vi "User Info.vi"(11 "User Entrence":string) -> ()   [LabVIEW 2020]
uses:
  <vilib>/addons/database/Connection.llb/Conn ObjectReference.ctl
  <vilib>/Utility/error.llb/whitespace.ctl
  <vilib>/addons/database/Connection.llb/DB Tools Open Connec (String).vi
  <vilib>/addons/database/Connection.llb/Conn Execute.vi
  <vilib>/addons/database/Recordset.llb/Rec Fetch Recordset Data (R).vi
  <vilib>/addons/database/Recordset.llb/Rec Destroy - Connection.vi
  <vilib>/addons/database/_DB Variant To Data/Database Variant To Data.xnode
  <vilib>/addons/database/NI_Database_API.lvlib
panel:
  in  "Back":bool
  in  "Tab Control":T1(tab)
  in  "User_Name 7":string caption="用户名"
  in  "User_Password 2":string caption="密    码"
  in  "Login":bool
  in  "Remember Passwrod":bool caption="记住密码"
  in  "Remember User Name":bool caption="记住用户名"
  in  "User Regist":bool
  in  "User Change":bool caption="切换用户"
  in  "User Manage":bool
  in  "Change Password":bool
  in  "User_Right 2":u16(ring) caption="权    限" items=["Manufacturer", "Foreman", "Professional", "Operator"]
  in  "User_Name 4":string caption="用户名"
  in  "Confirm Password 2":string caption="确认密码"
  in  "New Password 2":string caption="新  密  码"
  in  "Last Password":string caption="旧  密  码"
  in  "User Change Btn":bool
  in  "User_Name 3":string caption="用  户  名"
  in  "User_Password":string caption="密        码"
  in  "User_Name":string caption="用  户  名"
  in  "Ok":bool
  in  "User List":i32(listbox)
  in  "User_Right":u16(ring) caption="权        限" items=["Manufacturer", "Foreman", "Professional", "Operator"]
  in  "Confirm Password":string caption="确认密码"
  in  "New Password":string caption="密        码"
  in  "Ok 2":bool
  in  "User_Name 2":string caption="用  户  名"
  in  "User_Right 3":u16(ring) caption="权        限" items=["Manufacturer", "Foreman", "Professional", "Operator"]
  in  "Confirm Password 3":string caption="确认密码"
  in  "New Password 3":string caption="新  密  码"
  in  "Ok 4":bool
  in  "User_Name 5":string caption="用  户  名"
  in  "Confirm Password 4":string caption="确认密码"
  in  "New Password 4":string caption="密        码"
  in  "Regist":bool
  in  "User_Name 6":string caption="用  户  名"
  out "Title":string
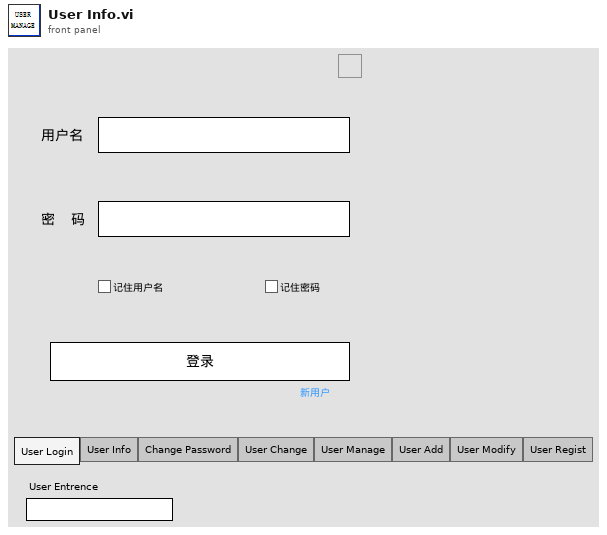
[diagram p1: front panel]
types:
  T1 = enum32{"User Login", "User Info", "Change Password", "User Change", "User Manage", "User Add", "User Modify", "User Regist"}
  T2 = typedef "NI_Database_API.lvlib/Conn ObjectReference.ctl" = refnum<k1>
  T3 = cluster{"DB Ref In":T2, "User Name":string, "User Password":string, "User Right":i32, "Language":string, "Current Page":string, "Tab Control":refnum<vi>, "Remember Name":bool, "Remember PW":bool}
  T4 = enum32{"Invalid", "Standard", "Closed", "Hidden", "Minimized", "Maximized"}
  T5 = cluster{"User Name":string, "User Right":i32, "User Password":string, string, string, "seconds since 1Jan1904":timestamp}
  T6 = typedef "whitespace.ctl" = u16
  T7 = typedef "NI_Database_API.lvlib/Rec ObjectReference.ctl" = refnum<k1>
  T8 = typedef "LVPoint32TypeDef.ctl" = cluster{"Horizontal":i32, "Vertical":i32}
  T9 = typedef "LVRowAndColumnTypeDef.ctl" = cluster{"Row":i32, "Column":i32}
  T10 = enum32{"invalid app kind", "Development System", "Run Time System", "Student Edition", "Embedded LabVIEW", "Evaluation", "Custom"}
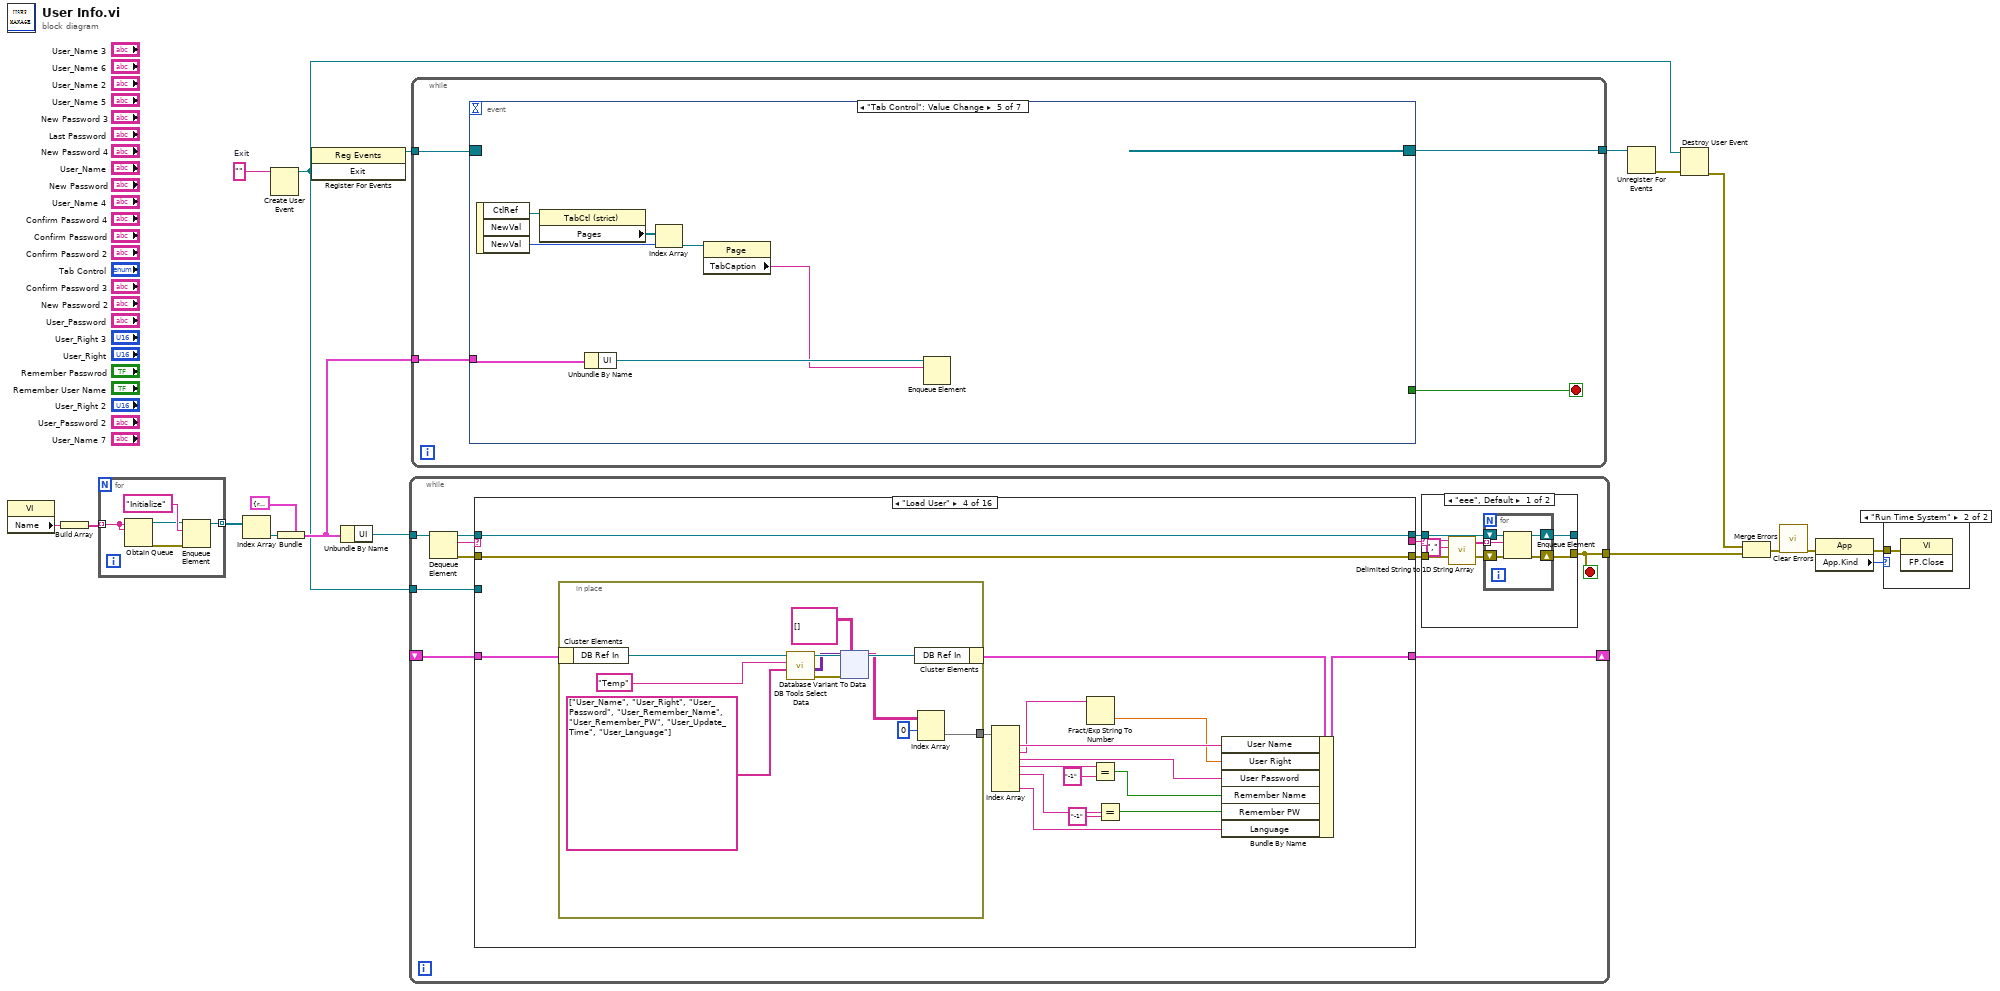
[diagram p0: block diagram]
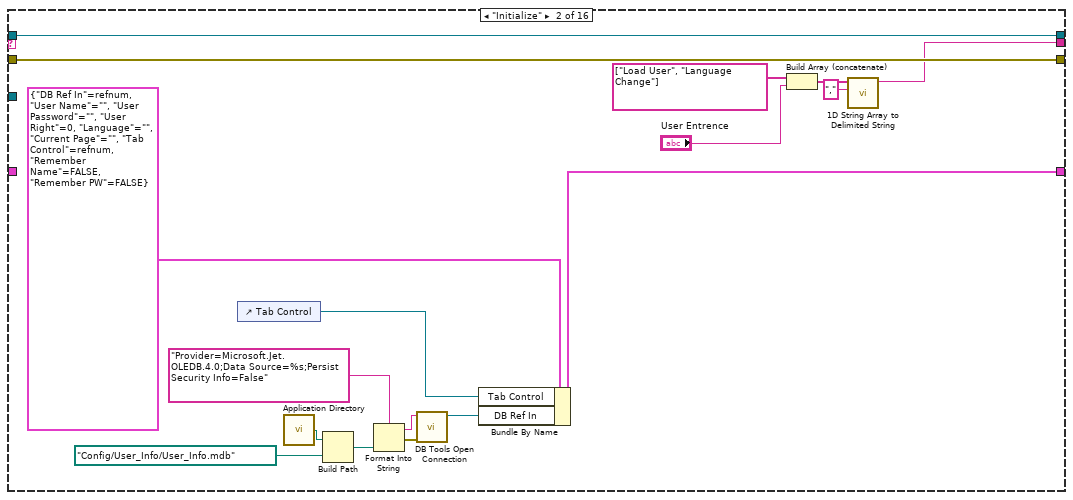
[diagram p5: hidden frame]
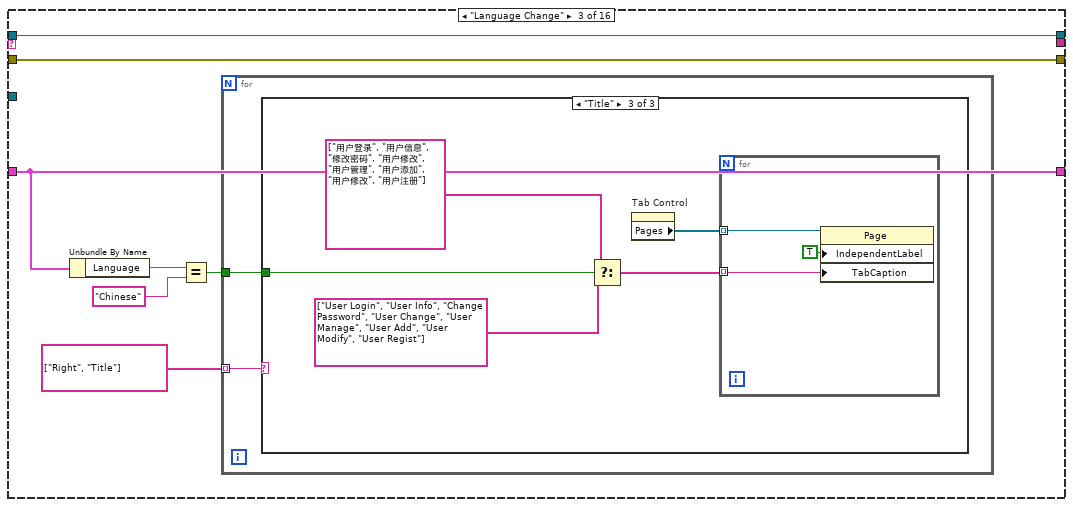
[diagram p6: hidden frame]
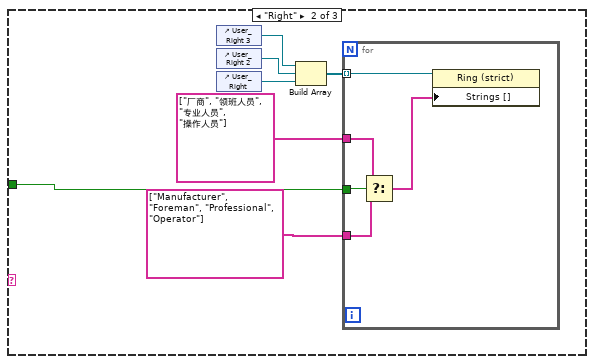
[diagram p8: hidden frame]
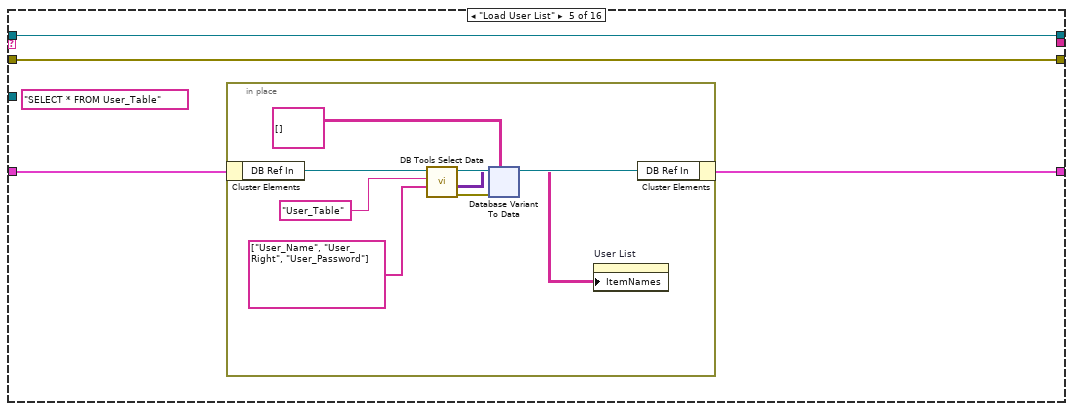
[diagram p9: hidden frame]
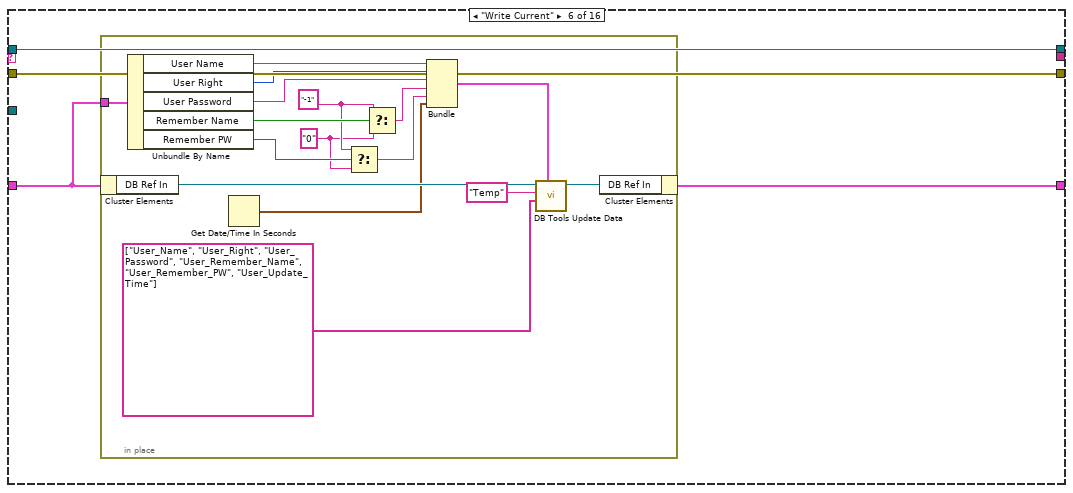
[diagram p10: hidden frame]
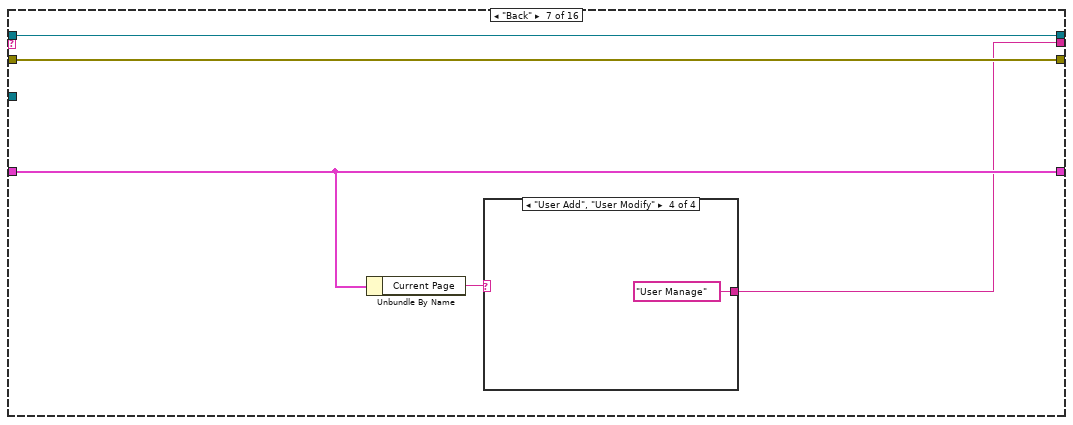
[diagram p11: hidden frame]
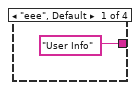
[diagram p12: hidden frame]
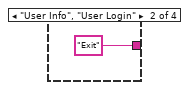
[diagram p13: hidden frame]
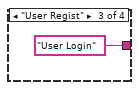
[diagram p14: hidden frame]
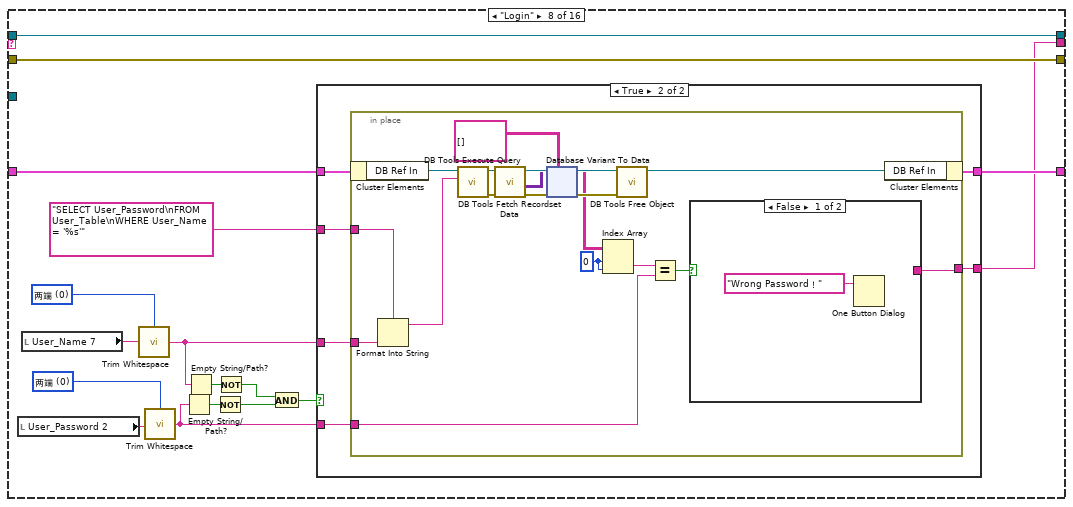
[diagram p15: hidden frame]
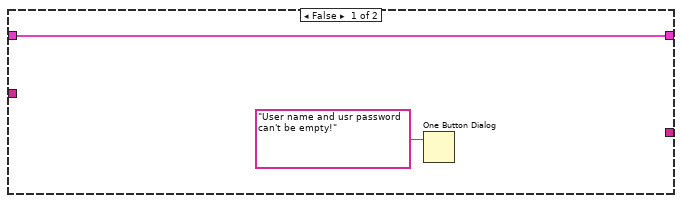
[diagram p16: hidden frame]
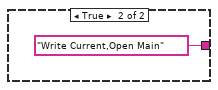
[diagram p17: hidden frame]
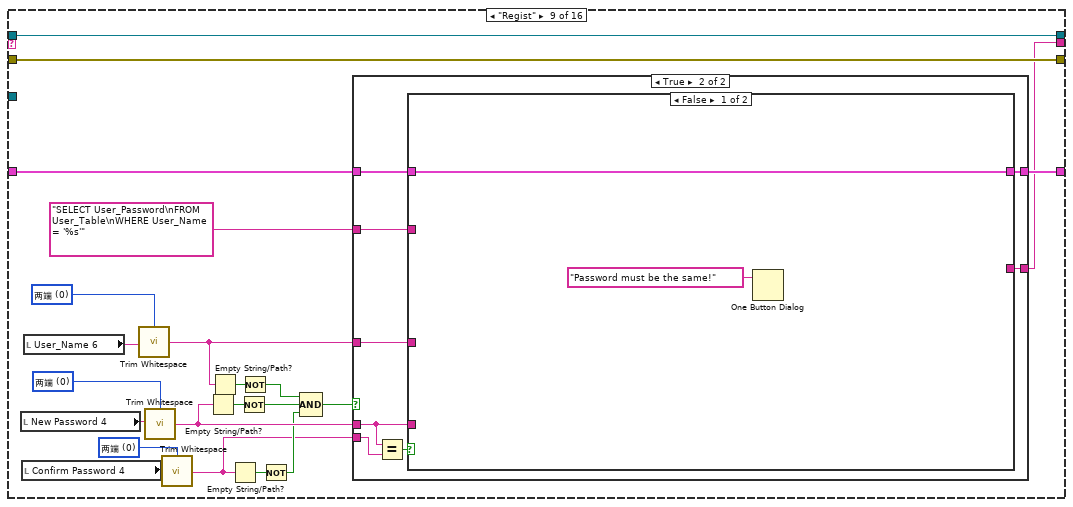
[diagram p18: hidden frame]
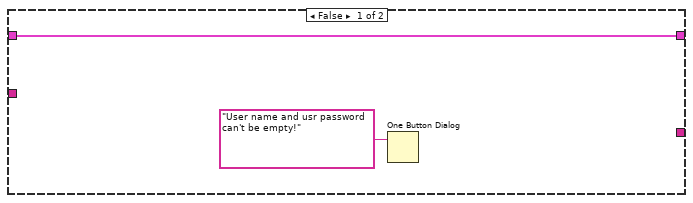
[diagram p19: hidden frame]
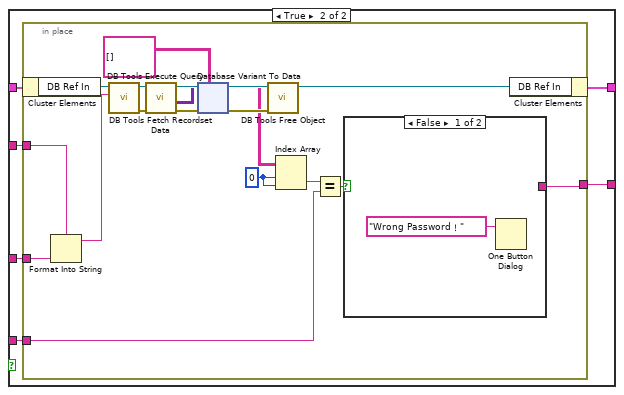
[diagram p20: hidden frame]
diagram:
  w3 = ""  # Exit
  n1 = property class="VI"() -> ("Name"=w13:string)  [unwired: 2 in, 2 out]
  n2 = Build Array(w13) -> (w14:string[])
  n3 = for {
    tunnel: w14 -> [w19] mode=indexing
    tunnel: [w20] -> w8 mode=indexing
    n4 = Obtain Queue(name (unnamed)=w19, element data type=w19) -> (queue out=w22:refnum<queue>, error out=w21:errorcluster)  [unwired: 3 in, 1 out]
    n5 = Enqueue Element(queue=w22, element="Initialize" ("元素"), error in (no error)=w21) -> (queue out=w20:refnum<queue>)  [unwired: 1 in, 2 out]
  }
  n6 = Index Array(array=w8) -> (element=w11:refnum<queue>)  [unwired: 1 in]
  n7 = Create User Event(user event datatype=w3) -> (user event=w7:refnum<user-event>)  [unwired: 1 in, 1 out]
  n8 = Bundle(cluster=cluster{"UI":refnum<queue>} {"UI"=refnum}, "UI"=w11) -> (w12:cluster{"UI":refnum<queue>})
  n9 = register-events(w7) -> (reference out=w4:refnum<event-registration>)  [unwired: 2 in, 1 out]
  n10 = Unbundle By Name(w12) -> ("UI"=w9:refnum<queue>)
  n11 = while {
    tunnel: w9 -> [w34]
    tunnel: [w24] -> w16
    shift-right: [w28] -> _
    shift-left: _ -> [w27]
    tunnel: w7 -> [w26]
    stop <- w24 stop-if-true
    n12 = Dequeue Element(queue=w34) -> (queue out=w33:refnum<queue>, element=w25:string, error out=w30:errorcluster)  [unwired: 2 in, 1 out]
    n13 = case shown="\"Load User\"" w25 {
      selector: w25 -> [_ _ _ _ _ _ _ _ _ _ _ _ _ w469 w524 _]
      tunnel: w33 -> [w51 w59 w75 w114 w172 w228 w249 w270 w364 w456 w459 w462 w465 w474 w529 w535]
      tunnel: [w51 w59 w75 w114 w172 w228 w249 w270 w364 w456 w459 w462 w465 w474 w528 w535] -> w32
      tunnel: [w50 w58 w74 w113 w171 w227 w248 w269 w363 w455 w458 w461 w464 w473 w527 w532] -> w31
      tunnel: w30 -> [w50 w58 w74 w113 w171 w227 w248 w269 w363 w455 w458 w461 w464 w473 w526 w534]
      tunnel: [_ w52 _ _ _ _ w245 w257 w352 "Exit" ("Message") _ _ _ w467 "Quit" ("Message") _] -> w29
      tunnel: [w49 w61 w73 w111 w169 w226 w247 w260 w354 w454 w457 w460 w463 w468 w531 w533] -> w28
      tunnel: w27 -> [w49 _ w73 w112 w170 w225 w247 w261 w355 w454 w457 w460 w463 w472 w531 w533]
      tunnel: w26 -> [_ _ _ _ _ _ _ _ _ _ _ _ _ _ w525 _]
      frame "eee", Default {
      }
      frame "Initialize" {
        n14 = control-ref of="Tab Control"() -> (w55:refnum<vi>)
        n15 = call <vilib>:"Application Directory.vi"() -> ("Application Directory"=w64:path)
        n16 = Build Path(base path=w64, name or relative path=path "Config/User_Info/User_Info.mdb" ("名称或相对路径")) -> (appended path=w62:path)
        n17 = Format Into String(format string="Provider=Microsoft.Jet.OLEDB.4.0;Data Source=%s;Persist Security Info=False", w62) -> (resulting string=w66:string, error out=w65:errorcluster)  [unwired: 2 in]
        n18 = call-poly <vilib>:"DB Tools Open Connection.vi"("error in (no error)"=w65, "connection information"=w66) -> ("connection reference"=w60:T2)  [unwired: 6 in, 1 out]
        n19 = Bundle By Name(cluster=T3 {"DB Ref In"=refnum, "User Name"="", "User Password"="", "User Right"=0, "Language"="", "Current Page"="", "Tab Control"=refnum, "Remember Name"=FALSE, "Remember PW"=FALSE} ("Data"), "Tab Control"=w55, "DB Ref In"=w60) -> (w61:T3)
        n20 = Build Array (concatenate)(string[] ["Load User", "Language Change"], "User Entrence") -> (w54:string[])
        n21 = call <vilib>:"1D String Array to Delimited String.vi"("delimiter"=",", "string array"=w54) -> ("delimited string"=w52:string)  [unwired: 9 in]
      }
      frame "Language Change" {
        n22 = Unbundle By Name(w73) -> ("Language"=w72:string)
        n23 = Equal?(x=w72, y="Chinese") -> (x = y?=w69:bool)
        n24 = for {
          tunnel: string[] ["Right", "Title"] -> [w77] mode=indexing
          tunnel: w69 -> [w76]
          n25 = case shown="\"Title\"" w77 {
            tunnel: w76 -> [_ w78 w94]
            frame "eee", Default {
            }
            frame "Right" {
              n26 = control-ref of="User_Right 3"() -> (w81:refnum<vi>)
              n27 = control-ref of="User_Right 2"() -> (w82:refnum<vi>)
              n28 = control-ref of="User_Right"() -> (w83:refnum<vi>)
              n29 = Build Array(w81, w82, w83) -> (w84:refnum<vi>[])
              n30 = for {
                tunnel: w84 -> [w89] mode=indexing
                tunnel: string[] ["厂商", "领班人员", "专业人员", "操作人员"] -> [w88]
                tunnel: string[] ["Manufacturer", "Foreman", "Professional", "Operator"] -> [w87]
                tunnel: w78 -> [w85]
                n31 = Select(t=w88, s=w85, f=w87) -> (s? t:f=w86:string[])
                n32 = property class="Ring (strict)"(reference=w89, "Strings []"=w86) -> ()  [unwired: 1 in, 2 out]
              }
            }
            frame "Title" {
              n33 = Select(t=string[] ["用户登录", "用户信息", "修改密码", "用户修改", "用户管理", "用户添加", "用户修改", "用户注册"], s=w94, f=string[] ["User Login", "User Info", "Change Password", "User Change", "User Manage", "User Add", "User Modify", "User Regist"]) -> (s? t:f=w90:string[])
              n34 = property on="Tab Control" class="TabCtl (strict)"() -> ("Pages"=w91:refnum<vi>[])  [unwired: 2 in, 2 out]
              n35 = for {
                tunnel: w91 -> [w97] mode=indexing
                tunnel: w90 -> [w96] mode=indexing
                n36 = property class="Page"(reference=w97, "IndependentLabel"=TRUE ("独立标签"), "TabCaption"=w96) -> ()  [unwired: 1 in, 2 out]
              }
            }
          }
        }
      }
      frame "Load User" {
        n37 = in-place {
          in-place-border: [w115] -> w109
          n38 = in-place-cluster #1(w112) -> ("DB Ref In"=w124:T2)
          n39 = call <vilib>:"DB Tools Select Data.vi"("columns"=string[] ["User_Name", "User_Right", "User_Password", "User_Remember_Name", "User_Remember_PW", "User_Update_Time", "User_Language"], "table"="Temp", "connection reference"=w124) -> ("error out"=w118:errorcluster, "data"=w120:variant[][], "connection reference out"=w123:T2)  [unwired: 3 in]
          n40 = xnode "Database Variant To Data"("database variant"=w120, "error in (no error)"=w118, "type"=string[][] []) -> ("data"=w117:string[][])  [unwired: 1 out]
          n41 = in-place-cluster #1("DB Ref In"=w123) -> (w110:T3)
          n42 = Index Array(array=w117, index (row)=0 ("索引 (行)")) -> (element=w115:string[])  [unwired: 1 in]
        }
        n43 = Index Array(array=w109) -> (element #1=w108:string, element #2=w99:string, element #3=w107:string, element #4=w106:string, element #5=w102:string, element #7=w100:string)  [unwired: 7 in, 1 out]
        n44 = Fract/Exp String To Number(string=w99) -> (number=w98:dbl)  [unwired: 3 in, 1 out]
        n45 = Equal?(x=w106, y="-1") -> (x = y?=w104:bool)
        n46 = Equal?(x=w102, y="-1") -> (x = y?=w101:bool)
        n47 = Bundle By Name(cluster=w110, "User Name"=w108, "User Right"=w98, "User Password"=w107, "Remember Name"=w104, "Remember PW"=w101, "Language"=w100) -> (w111:T3)
      }
      frame "Load User List" {
        (unwired) "SELECT * FROM User_Table" ("SQL query")
        n48 = in-place {
          n49 = in-place-cluster #2(w170) -> ("DB Ref In"=w180:T2)
          n50 = call <vilib>:"DB Tools Select Data.vi"("columns"=string[] ["User_Name", "User_Right", "User_Password"] ("table"), "table"="User_Table", "connection reference"=w180) -> ("error out"=w176:errorcluster, "data"=w175:variant[][], "connection reference out"=w179:T2)  [unwired: 3 in]
          n51 = xnode "Database Variant To Data"("database variant"=w175, "error in (no error)"=w176, "type"=string[][] []) -> ("data"=w173:string[][])  [unwired: 1 out]
          n52 = property on="User List" class="MCListbox (strict)"("ItemNames"=w173) -> ()  [unwired: 2 in, 2 out]
          n53 = in-place-cluster #2("DB Ref In"=w179) -> (w169:T3)
        }
      }
      frame "Write Current" {
        n54 = in-place {
          in-place-border: w225 -> [w241]
          w230 = "0"
          w231 = "-1"
          n55 = in-place-cluster #3(w225) -> ("DB Ref In"=w244:T2)
          n56 = Unbundle By Name(w241) -> ("User Name"=w240:string, "User Right"=w239:i32, "User Password"=w238:string, "Remember Name"=w235:bool, "Remember PW"=w233:bool)
          n57 = Get Date/Time In Seconds() -> (seconds since 1Jan1904=w229:timestamp)
          n58 = Select(t=w231, s=w233, f=w230) -> (s? t:f=w232:string)
          n59 = Select(t=w231, s=w235, f=w230) -> (s? t:f=w234:string)
          n60 = Bundle("User Name"=w240, "User Right"=w239, "User Password"=w238, w234, w232, "seconds since 1Jan1904"=w229) -> (w237:T5)  [unwired: 1 in]
          n61 = call <vilib>:"DB Tools Update Data.vi"("data"=w237, "columns"=string[] ["User_Name", "User_Right", "User_Password", "User_Remember_Name", "User_Remember_PW", "User_Update_Time"], "table"="Temp", "connection reference"=w244) -> ("connection reference out"=w243:T2)  [unwired: 6 in, 1 out]
          n62 = in-place-cluster #3("DB Ref In"=w243) -> (w226:T3)
        }
      }
      frame "Back" {
        n63 = Unbundle By Name(w247) -> ("Current Page"=w246:string)
        n64 = case shown="\"User Add\", \"User Modify\"" w246 {
          tunnel: ["User Info" "Exit" "User Login" "User Manage"] -> w245
          frame "eee", Default {
          }
          frame "User Info", "User Login" {
          }
          frame "User Regist" {
          }
          frame "User Add", "User Modify" {
          }
        }
      }
      frame "Login" {
        w267 = T6 0 items=["两端", "字符串首端", "字符串末端"] ("location (both)")
        w268 = T6 0 items=["两端", "字符串首端", "字符串末端"] ("location (both)")
        n65 = local read "User_Password 2"() -> (w254:string)
        n66 = local read "User_Name 7"() -> (w255:string)
        n67 = call <vilib>:"Trim Whitespace.vi"("string"=w255, "location (both)"=w268) -> ("trimmed string"=w259:string)
        n68 = call <vilib>:"Trim Whitespace.vi"("string"=w254, "location (both)"=w267) -> ("trimmed string"=w258:string)
        n69 = Empty String/Path?(string/path=w258) -> (empty?=w265:bool)
        n70 = Empty String/Path?(string/path=w259) -> (empty?=w266:bool)
        n71 = Not(x=w265) -> (.not. x?=w264:bool)
        n72 = Not(x=w266) -> (.not. x?=w263:bool)
        n73 = And(x=w263, y=w264) -> (x .and. y?=w262:bool)
        n74 = case shown="True" w262 {
          tunnel: w261 -> [w271 w278]
          tunnel: [w271 w277] -> w260
          tunnel: w259 -> [_ w276]
          tunnel: w258 -> [_ w275]
          tunnel: [_ w274] -> w257
          tunnel: "SELECT User_Password\nFROM User_Table\nWHERE User_Name = '%s'" ("SQL query") -> [_ w273]
          frame False {
            n75 = One Button Dialog(message="User name and usr password can't be empty!" ("消息")) -> ()  [unwired: 1 in, 1 out]
          }
          frame True {
            n76 = in-place {
              in-place-border: w276 -> [w286]
              in-place-border: w275 -> [w282]
              in-place-border: [w279] -> w274
              in-place-border: w273 -> [w281]
              w284 = 0 ("索引 (行)")
              n77 = in-place-cluster #4(w278) -> ("DB Ref In"=w288:T2)
              n78 = Format Into String(format string=w281, w286) -> (resulting string=w290:string)  [unwired: 2 in, 1 out]
              n79 = call-poly <vilib>:"DB Tools Execute Query.vi"("SQL query"=w290, "connection reference"=w288) -> ("error out"=w295:errorcluster, "recordset reference"=w293:T7)  [unwired: 6 in]
              n80 = call-poly <vilib>:"DB Tools Fetch Recordset Data.vi"("error in (no error)"=w295, "recordset reference"=w293) -> ("error out"=w291:errorcluster, "recordset data"=w292:variant[][], "recordset reference out"=w294:T7)  [unwired: 3 in]
              n81 = xnode "Database Variant To Data"("database variant"=w292, "error in (no error)"=w291, "type"=string[][] []) -> ("data"=w285:string[][], "error out"=w296:errorcluster)
              n82 = Index Array(array=w285, index (row)=w284, index (col)=w284) -> (element=w283:string)
              n83 = call-poly <vilib>:"DB Tools Free Object.vi"("error in (no error)"=w296, "recordset reference"=w294) -> ("connection reference"=w287:T2)  [unwired: 8 in, 1 out]
              n84 = Equal?(x=w283, y=w282) -> (x = y?=w280:bool)
              n85 = case shown="False" w280 {
                tunnel: [_ "Write Current,Open Main"] -> w279
                frame False {
                  n86 = One Button Dialog(message="Wrong Password！" ("消息")) -> ()  [unwired: 1 in, 1 out]
                }
                frame True {
                }
              }
              n87 = in-place-cluster #4("DB Ref In"=w287) -> (w277:T3)
            }
          }
        }
      }
      frame "Regist" {
        w346 = T6 0 items=["两端", "字符串首端", "字符串末端"] ("location (both)")
        w361 = T6 0 items=["两端", "字符串首端", "字符串末端"] ("location (both)")
        w362 = T6 0 items=["两端", "字符串首端", "字符串末端"] ("location (both)")
        n88 = local read "New Password 4"() -> (w349:string)
        n89 = local read "Confirm Password 4"() -> (w347:string)
        n90 = local read "User_Name 6"() -> (w350:string)
        n91 = call <vilib>:"Trim Whitespace.vi"("string"=w350, "location (both)"=w362) -> ("trimmed string"=w353:string)
        n92 = call <vilib>:"Trim Whitespace.vi"("string"=w349, "location (both)"=w361) -> ("trimmed string"=w348:string)
        n93 = call <vilib>:"Trim Whitespace.vi"("string"=w347, "location (both)"=w346) -> ("trimmed string"=w343:string)
        n94 = Empty String/Path?(string/path=w348) -> (empty?=w359:bool)
        n95 = Empty String/Path?(string/path=w353) -> (empty?=w360:bool)
        n96 = Empty String/Path?(string/path=w343) -> (empty?=w345:bool)
        n97 = Not(x=w359) -> (.not. x?=w358:bool)
        n98 = Not(x=w360) -> (.not. x?=w357:bool)
        n99 = Not(x=w345) -> (.not. x?=w344:bool)
        n100 = Compound Arithmetic op=AND ("复合运算")(w357, w358, w344) -> (w356:bool)
        n101 = case shown="True" w356 {
          tunnel: w355 -> [w365 w374]
          tunnel: [w365 w373] -> w354
          tunnel: w353 -> [_ w372]
          tunnel: w348 -> [_ w369]
          tunnel: [_ w371] -> w352
          tunnel: "SELECT User_Password\nFROM User_Table\nWHERE User_Name = '%s'" ("SQL query") -> [_ w370]
          tunnel: w343 -> [_ w368]
          frame False {
            n102 = One Button Dialog(message="User name and usr password can't be empty!" ("消息")) -> ()  [unwired: 1 in, 1 out]
          }
          frame True {
            n103 = Equal?(x=w369, y=w368) -> (x = y?=w367:bool)
            n104 = case shown="False" w367 {
              tunnel: w374 -> [w376 w382]
              tunnel: [w376 w381] -> w373
              tunnel: w372 -> [_ w380]
              tunnel: [_ w379] -> w371
              tunnel: w370 -> [_ w378]
              tunnel: w369 -> [_ w377]
              frame False {
                n105 = One Button Dialog(message="Password must be the same!" ("消息")) -> ()  [unwired: 1 in, 1 out]
              }
              frame True {
                n106 = in-place {
                  in-place-border: w380 -> [w390]
                  in-place-border: w377 -> [w386]
                  in-place-border: [w383] -> w379
                  in-place-border: w378 -> [w385]
                  w388 = 0 ("索引 (行)")
                  n107 = in-place-cluster #5(w382) -> ("DB Ref In"=w392:T2)
                  n108 = Format Into String(format string=w385, w390) -> (resulting string=w394:string)  [unwired: 2 in, 1 out]
                  n109 = call-poly <vilib>:"DB Tools Execute Query.vi"("SQL query"=w394, "connection reference"=w392) -> ("error out"=w399:errorcluster, "recordset reference"=w397:T7)  [unwired: 6 in]
                  n110 = call-poly <vilib>:"DB Tools Fetch Recordset Data.vi"("error in (no error)"=w399, "recordset reference"=w397) -> ("error out"=w395:errorcluster, "recordset data"=w396:variant[][], "recordset reference out"=w398:T7)  [unwired: 3 in]
                  n111 = xnode "Database Variant To Data"("database variant"=w396, "error in (no error)"=w395, "type"=string[][] []) -> ("data"=w389:string[][], "error out"=w400:errorcluster)
                  n112 = call-poly <vilib>:"DB Tools Free Object.vi"("error in (no error)"=w400, "recordset reference"=w398) -> ("connection reference"=w391:T2)  [unwired: 8 in, 1 out]
                  n113 = Index Array(array=w389, index (row)=w388, index (col)=w388) -> (element=w387:string)
                  n114 = Equal?(x=w387, y=w386) -> (x = y?=w384:bool)
                  n115 = case shown="False" w384 {
                    tunnel: [_ "Write Current,Open Main"] -> w383
                    frame False {
                      n116 = One Button Dialog(message="Wrong Password！" ("消息")) -> ()  [unwired: 1 in, 1 out]
                    }
                    frame True {
                    }
                  }
                  n117 = in-place-cluster #5("DB Ref In"=w391) -> (w381:T3)
                }
              }
            }
          }
        }
      }
      frame "Open Main" {
        n118 = vi-ref "Device_Connect.vi"() -> (w453:refnum<vi>)
        n119 = invoke class="VI" method="FP.Open"(reference=w453, "Activate"=TRUE ("激活？"), "State"=T4."Standard" ("状态")) -> (reference out=w452:refnum<vi>)  [unwired: 2 in, 4 out]
        n120 = invoke class="VI" method="Run VI"(reference=w452, "Wait until done"=FALSE ("结束前等待"), "Auto Dispose Ref"=FALSE ("自动销毁引用")) -> ()  [unwired: 2 in, 5 out]
      }
      frame "====Change Password====" {
      }
      frame "====User Change====" {
      }
      frame "User Change Btn" {
      }
      frame "Change Password", "User Add", "User Change", "User Info", "User Login", "User Manage", "User Modify", "User Regist" {
        n121 = property on="Tab Control" class="TabCtl (strict)"() -> ("Pages"=w471:refnum<vi>[])  [unwired: 2 in, 2 out]
        n122 = Bundle By Name(cluster=w472, "Current Page"=w469) -> (w468:T3)
        n123 = for {
          tunnel: w471 -> [w523] mode=indexing
          tunnel: w469 -> [w521]
          tunnel: [w519] -> w470
          tunnel: [w518] -> w466
          i -> [w519]
          stop <- w520 stop-if-true
          n124 = property class="Page"(reference=w523) -> ("PageLabel"=w522:string, "TabCaption"=w518:string)  [unwired: 1 in, 2 out]
          n125 = Equal?(x=w521, y=w522) -> (x = y?=w520:bool)
        }
        "Title" <- w466
        n126 = property on="Tab Control" class="TabCtl (strict)"("Value"=w470) -> ()  [unwired: 2 in, 2 out]
        n127 = property class="VI"("Front Panel.Title"=w466) -> ()  [unwired: 2 in, 2 out]
        n128 = case shown="\"User Info\"" w469 {
          tunnel: w468 -> [_ w483 _ _ w509 _ _ w517]
          tunnel: [_ _ _ "Load User List" _ _ _ _] -> w467
          frame "eee", Default {
          }
          frame "User Login" {
            n129 = Unbundle By Name(w483) -> ("User Name"=w480:string, "User Password"=w481:string, "Remember Name"=w482:bool, "Remember PW"=w479:bool)
            n130 = case shown="True" w482 {
              selector: w482 -> [w484 w487]
              tunnel: w481 -> [_ w491]
              tunnel: w480 -> [_ w492]
              tunnel: w479 -> [w485 w493]
              tunnel: [_ w490] -> w478
              tunnel: [_ w489] -> w477
              tunnel: [w485 w488] -> w475
              tunnel: [w484 w486] -> w476
              frame False {
              }
              frame True {
                n131 = case shown="True" w493 {
                  selector: w493 -> [w495 w497]
                  tunnel: w492 -> [w496 w500]
                  tunnel: w491 -> [_ w499]
                  tunnel: [w496 w500] -> w490
                  tunnel: [_ w499] -> w489
                  tunnel: [w495 w497] -> w488
                  tunnel: w487 -> [w494 w498]
                  tunnel: [w494 w498] -> w486
                  frame False {
                  }
                  frame True {
                  }
                }
              }
            }
            n132 = local write "User_Name 7"(w478) -> ()
            n133 = local write "User_Password 2"(w477) -> ()
            n134 = local write "Remember User Name"(w476) -> ()
            n135 = local write "Remember Passwrod"(w475) -> ()
          }
          frame "User Regist" {
            n136 = local write "Confirm Password 4"("" ("Confirm Password 4")) -> ()
            n137 = local write "New Password 4"("" ("New Password 4")) -> ()
            n138 = local write "User_Name 6"("" ("User_Name 6")) -> ()
          }
          frame "User Manage" {
          }
          frame "Change Password" {
            n139 = Unbundle By Name(w509) -> ("User Name"=w508:string)
            n140 = local write "User_Name 3"(w508) -> ()
            n141 = local write "Last Password"("" ("Last Password")) -> ()
            n142 = local write "New Password 2"("" ("New Password 2")) -> ()
            n143 = local write "Confirm Password 2"("" ("Confirm Password 2")) -> ()
          }
          frame "User Change" {
            n144 = local write "User_Name"("" ("User_Name")) -> ()
            n145 = local write "User_Password"("" ("User_Password")) -> ()
          }
          frame "User Add" {
            n146 = local write "User_Name 2"("" ("User_Name 2")) -> ()
            n147 = local write "New Password"("" ("New Password")) -> ()
            n148 = local write "Confirm Password"("" ("Confirm Password")) -> ()
          }
          frame "User Info" {
            n149 = Unbundle By Name(w517) -> ("User Name"=w516:string, "User Right"=w515:i32)
            n150 = local write "User_Name 4"(w516) -> ()
            n151 = local write "User_Right 2"(w515) -> ()
          }
        }
      }
      frame "Exit" {
        n152 = Generate User Event(user event=w525, event data cluster=w524) -> ()  [unwired: 2 in, 2 out]
        n153 = Flush Queue(queue=w529, error in (no error)=w526) -> (queue out=w528:refnum<queue>, error out=w527:errorcluster)  [unwired: 1 out]
      }
      frame "Quit" {
        n154 = Release Queue(queue=w535, error in (no error)=w534) -> (error out=w532:errorcluster)  [unwired: 1 in, 2 out]
      }
    }
    n155 = case shown="\"eee\", Default" w29 {
      selector: w29 -> [w37 _]
      tunnel: w32 -> [w41 w48]
      tunnel: w31 -> [w40 w47]
      tunnel: [w39 w47] -> w24
      tunnel: [w38 w48] -> _
      frame "eee", Default {
        n156 = call <vilib>:"Delimited String to 1D String Array.vi"("delimiter"=",", "delimited string"=w37) -> ("string array"=w35:string[])  [unwired: 9 in]
        n157 = for {
          shift-right: [w43] -> w38
          shift-left: w41 -> [w46]
          shift-right: [w44] -> w39
          shift-left: w40 -> [w45]
          tunnel: w35 -> [w42] mode=indexing
          n158 = Enqueue Element(queue=w46, element=w42, error in (no error)=w45) -> (queue out=w43:refnum<queue>, error out=w44:errorcluster)  [unwired: 1 in, 1 out]
        }
      }
      frame "" {
      }
    }
  }
  n159 = while {
    tunnel: w4 -> [w538]
    tunnel: [w537] -> w6
    tunnel: w12 -> [w536]
    stop <- w539 stop-if-true
    n160 = event shown="[4] \"Tab Control\": Value Change" {
      selector: w538 -> [_ _ _ _ _ _ _]
      dyn-events: [_ _ _ _ _ _ _] -> w537
      timeout: _ -> [_ _ _ _ _ _ _]
      tunnel: [_ w541 _ _ _ _ _] -> w539
      tunnel: w536 -> [_ _ _ w548 w553 w561 w568]
      event Timeout {
        n161 = event-data() -> ()  [unwired: 1 in, 1 out]
      }
      event User Event {
        n162 = event-data() -> ("Exit"=w542:string)  [unwired: 1 in]
        n163 = Equal?(x=w542, y="Exit") -> (x = y?=w541:bool)
      }
      event Key Down {
        n164 = event-data() -> ("Char"=w544:i16, "PlatMods.Ctrl"=w543:bool)  [unwired: 1 in]
        n165 = case shown="True" w543 {
          tunnel: w544 -> [_ w545]
          frame False {
          }
          frame True {
            n166 = case shown="101" w545 {
              frame 0, Default {
              }
              frame 101 {
                n167 = property class="VI"("BDWin.Open"=TRUE ("程序框图窗口:打开")) -> ()  [unwired: 2 in, 2 out]
              }
            }
          }
        }
      }
      event Panel Close? {
        n168 = event-data() -> ()  [unwired: 1 in, 1 out]
        n169 = Unbundle By Name(w548) -> ("UI"=w547:refnum<queue>)
        n170 = Enqueue Element(queue=w547, element="Back" ("元素")) -> ()  [unwired: 2 in, 3 out]
        n171 = event-data("Discard?"=TRUE ("放弃？")) -> ()  [unwired: 1 in, 1 out]
      }
      event "Tab Control": Value Change {
        n172 = event-data() -> ("CtlRef"=w557:refnum<vi>, "NewVal"=w556:T1)  [unwired: 1 in, 1 out]
        n173 = property class="TabCtl (strict)"(reference=w557) -> ("Pages"=w555:refnum<vi>[])  [unwired: 1 in, 2 out]
        n174 = Unbundle By Name(w553) -> ("UI"=w552:refnum<queue>)
        n175 = Index Array(array=w555, index=w556) -> (element=w554:refnum<vi>)
        n176 = property class="Page"(reference=w554) -> ("TabCaption"=w551:string)  [unwired: 1 in, 2 out]
        n177 = Enqueue Element(queue=w552, element=w551) -> ()  [unwired: 2 in, 3 out]
      }
      event "Change Password", "User Change", "User Manage", "Back", "User Regist", "Login", "User Change Btn", "Ok", "Ok 2", "Ok 4", "Regist": Value Change {
        n178 = event-data() -> ("CtlRef"=w559:refnum<vi>)  [unwired: 1 in]
        n179 = Unbundle By Name(w561) -> ("UI"=w560:refnum<queue>)
        n180 = property class="Bool"(reference=w559) -> ("Label.Text"=w558:string)  [unwired: 1 in, 2 out]
        n181 = Enqueue Element(queue=w560, element=w558) -> ()  [unwired: 2 in, 3 out]
      }
      event "User List": Double Click {
        n182 = event-data() -> ("CtlRef"=w570:refnum<vi>, "Coords"=w569:T8)  [unwired: 1 in, 1 out]
        n183 = invoke class="MCListbox (strict)" method="Point To Row Column"(reference=w570, "Point"=w569) -> (reference out=w571:refnum<vi>, "InBounds"=w572:bool, "CellPosition"=w563:T9)  [unwired: 5 in, 4 out]
        n184 = property class="MCListbox (strict)"(reference=w571) -> (reference out=w565:refnum<vi>, "ItemNames"=w564:string[][])  [unwired: 1 in, 1 out]
        n185 = Matrix Size(0:w564) -> (1:w566:i32)  [unwired: 1 out]
        n186 = Unbundle(w563) -> ("Row"=w567:i32)  [unwired: 1 out]
        n187 = Less?(x=w566, y=w567) -> (x < y?=w562:bool)
        n188 = case shown="False" w572 {
          tunnel: w563 -> [_ w579]
          tunnel: w565 -> [_ w580]
          tunnel: w568 -> [_ w578]
          tunnel: w562 -> [_ w576]
          frame False {
          }
          frame True {
            n189 = property class="MCListbox (strict)"(reference=w580, "ActiveCell"=w579) -> ()  [unwired: 1 in, 2 out]
            n190 = Select(t="User Add" ("元素"), s=w576, f="User Modify" ("元素")) -> (s? t:f=w573:string)
            n191 = Unbundle By Name(w578) -> ("UI"=w577:refnum<queue>)
            n192 = Enqueue Element(queue=w577, element=w573) -> ()  [unwired: 2 in, 3 out]
          }
        }
      }
    }
  }
  n193 = Unregister For Events(event registration refnum=w6) -> (error out=w5:errorcluster)  [unwired: 1 in]
  n194 = Destroy User Event(user event=w7, error in=w5) -> (error out=w15:errorcluster)
  n195 = Merge Errors(w15, w16) -> (w17:errorcluster)
  n196 = call <vilib>:"Clear Errors.vi"("error in (no error)"=w17) -> ("error out"=w18:errorcluster)  [unwired: 5 in, 1 out]
  n197 = property class="App"(error in=w18) -> (error out=w1:errorcluster, "App.Kind"=w2:T10)  [unwired: 1 in, 1 out]
  n198 = case shown="\"Run Time System\"" w2 {
    tunnel: w1 -> [_ w581]
    frame "invalid app kind", Default {
    }
    frame "Run Time System" {
      n199 = invoke class="VI" method="FP.Close"(error in=w581) -> ()  [unwired: 2 in, 3 out]
    }
  }
